vi "From Variant.vi"(0 "Obj in":refnum<class "SAM.lvclass">, 7 "Variant":variant, 9 "Prefix":string, 11 "error in (no error)":errorcluster) -> (4 "Obj out":refnum<class "SAM.lvclass">, 15 "error out":errorcluster)   [LabVIEW 2020, in "SAM.lvclass"]
uses:
  SAM.lvclass
  SAM.lvclass/SAM.ctl
  AM/AM.lvclass
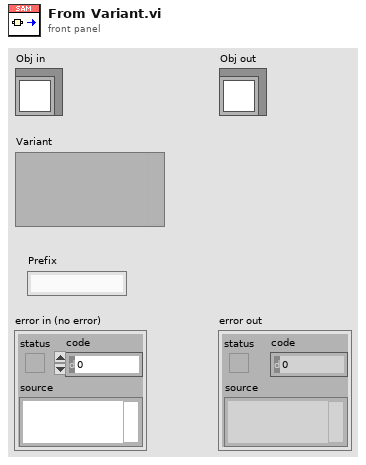
[diagram p1: front panel]
types:
  T1 = typedef "SAM.lvclass/Serialized.ctl" = cluster{"Frequency (Hz)":dbl, "Phase (0-1)":dbl}
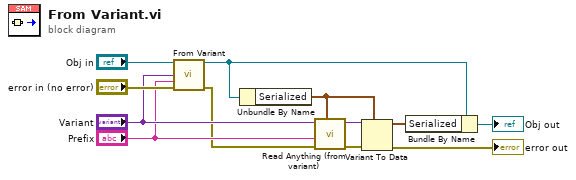
[diagram p0: block diagram]
diagram:
  n1 = call-parent "From Variant.vi"("Obj in"="Obj in", "Variant"="Variant", "Prefix"="Prefix", "error in (no error)"="error in (no error)") -> ("Obj out"=w3:refnum<class "SAM.lvclass">, "error out"=w4:errorcluster)  [unwired: 10 in]
  n2 = Unbundle By Name(w3) -> ("Serialized"=w8:T1)
  n3 = call "Read Anything (from variant).vi"("Type of Anything"=w8, "Error In"=w4, "Prefix"="Prefix", "Variant Database"="Variant") -> ("Error Out"=w9:errorcluster, "Anything"=w10:variant)  [unwired: 5 in, 1 out]
  n4 = Variant To Data(error in=w9, type=w8, Variant=w10) -> (data=w7:T1, error out=→"error out":errorcluster)
  n5 = Bundle By Name(cluster=w3, "Serialized"=w7) -> (→"Obj out":refnum<class "SAM.lvclass">)
